vi "Close.vi"(8 "error in (no error)":errorcluster, 11 "PSU_N87 in":refnum<class "PSU_N87.lvclass">) -> (0 "error out":errorcluster)   [LabVIEW 2014, in "PSU_N87.lvclass"]
uses:
  PSU_N87.lvclass
  PSU_N87.lvclass/PSU_N87.ctl
  data/Agilent N87XX Series.lvlib
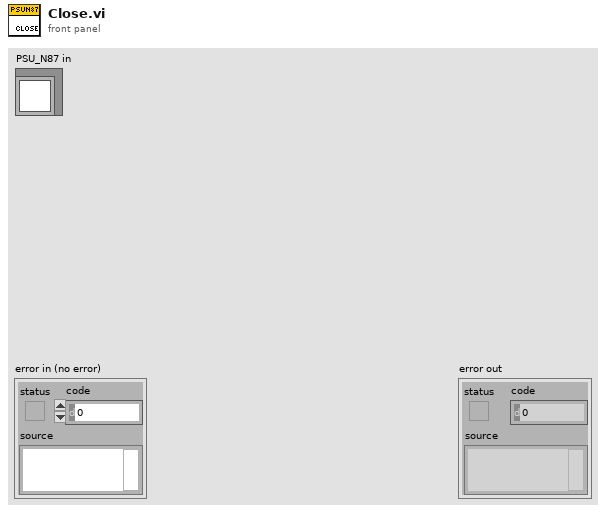
[diagram p1: front panel]
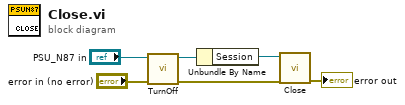
[diagram p0: block diagram]
diagram:
  n1 = call-dynamic "TurnOff.vi"("error in (no error)"="error in (no error)", "PSU_N87 in"="PSU_N87 in") -> ("error out"=w1:errorcluster, "PSU_N87 out"=w4:refnum<class "PSU_N87.lvclass">)  [unwired: 8 in]
  n2 = Unbundle By Name(w4) -> ("Session"=w2:refnum<visa-resource-name>)
  n3 = call "Close.vi"("error in (no error)"=w1, "VISA resource name"=w2) -> ("error out"=→"error out":errorcluster)  [unwired: 9 in]
